vi "GEN_User Login Verify.vi"(8 "error in":errorcluster caption="错误输入（无错误）", 11 "User Archives":T1={"User Archives"=[{"User Name"="Admin", "Code"="123456", "Ability"=enum."Administrator", "Last Log Time"=timestamp(3476160307.20119 s since 1904-01-01)}, {"User Name"="Liusj", "Code"="123456", "Ability"=enum."Operator", "Last Log Time"=timestamp(3476160734.0536046 s since 1904-01-01)}], "Current User"=-1}) -> (0 "error out":errorcluster caption="错误输出", 1 "User Exist?":bool, 2 "User Archives out":T1={"User Archives"=[{"User Name"="Admin", "Code"="123456", "Ability"=enum."Administrator", "Last Log Time"=timestamp(3476160307.20119 s since 1904-01-01)}, {"User Name"="Liusj", "Code"="123456", "Ability"=enum."Operator", "Last Log Time"=timestamp(3476160734.0536046 s since 1904-01-01)}], "Current User"=-1}, 4 "Cancel?":bool)   [LabVIEW 2016]
uses:
  User Login_Archives Data Structure.ctl
panel:
  in  "Cancel Login":bool
  in  "User Login":bool
  in  "Code":string caption="密  码"
  in  "User Name":string="Admin" caption="用户名"
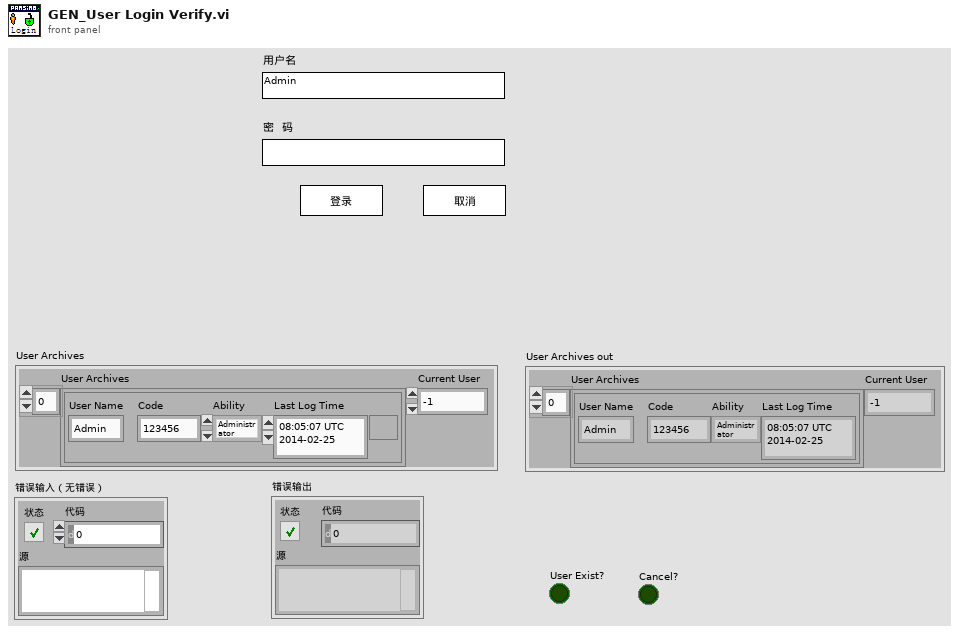
[diagram p1: front panel]
types:
  T1 = typedef "User Login_Archives Data Structure.ctl" = cluster{"User Archives":cluster{"User Name":string, "Code":string, "Ability":enum16{"Administrator", "Operator"}, "Last Log Time":timestamp}[], "Current User":i32}
  T2 = enum32{"Invalid", "Standard", "Closed", "Hidden", "Minimized", "Maximized"}
  T3 = cluster{"User Name":string, "Code":string, "Ability":enum16{"Administrator", "Operator"}, "Last Log Time":timestamp}[]
  T4 = cluster{"User Name":string, "Code":string, "Ability":enum16{"Administrator", "Operator"}, "Last Log Time":timestamp}
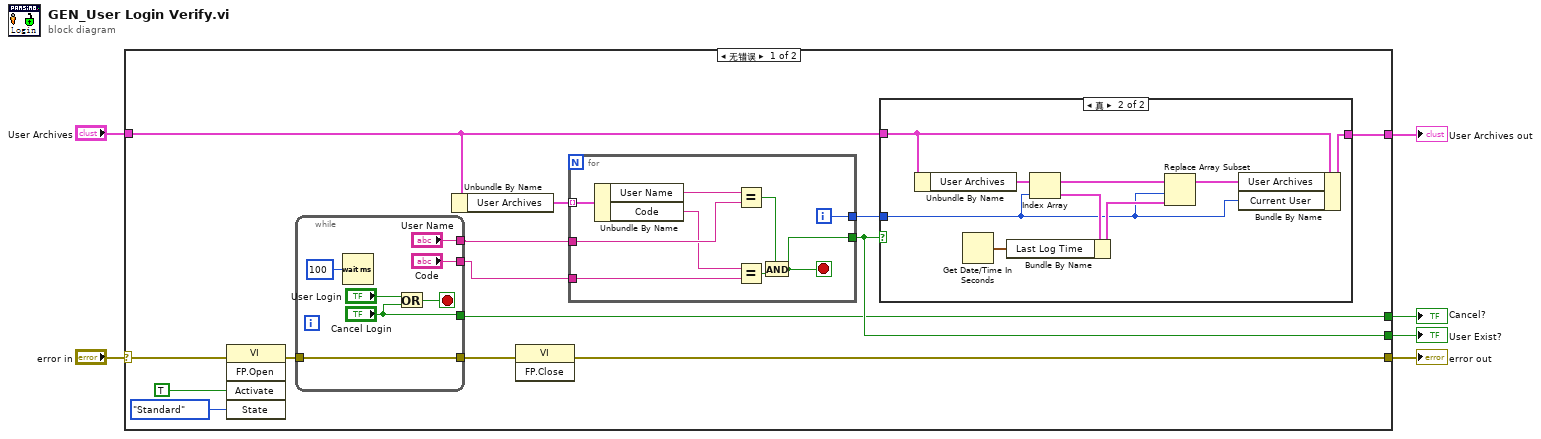
[diagram p0: block diagram]
diagram:
  n1 = case shown="无错误" "error in" {
    selector: "error in" -> [w13 w46]
    tunnel: [w19 _] -> w6
    tunnel: "User Archives" -> [w18 w47]
    tunnel: [w16 w47] -> w4
    tunnel: [w7 w46] -> w2
    tunnel: [w12 _] -> w1
    frame No Error {
      n2 = invoke class="VI" method="FP.Open"(error in=w13, "Activate"=TRUE ("激活？"), "State"=T2."Standard" ("状态")) -> (error out=w9:errorcluster)  [unwired: 2 in, 4 out]
      n3 = while {
        tunnel: ["User Name"] -> w15
        tunnel: ["Code"] -> w14
        tunnel: ["Cancel Login"] -> w12
        tunnel: w9 -> [w21]
        tunnel: [w21] -> w8
        stop <- w24 stop-if-true
        n4 = Wait (ms) ("等待(ms)")(milliseconds to wait=u32 100 ("等待时间（毫秒）")) -> ()  [unwired: 1 out]
        n5 = Or(x="User Login", y="Cancel Login") -> (x .or. y?=w24:bool)
      }
      n6 = Unbundle By Name(w18) -> ("User Archives"=w20:T3)
      n7 = invoke class="VI" method="FP.Close"(error in=w8) -> (error out=w7:errorcluster)  [unwired: 2 in, 2 out]
      n8 = for {
        tunnel: w15 -> [w43]
        tunnel: w14 -> [w41]
        tunnel: w20 -> [w45] mode=indexing
        tunnel: [w38] -> w19
        tunnel: [w37] -> w17
        i -> [w37]
        stop <- w38 stop-if-true
        n9 = Unbundle By Name(w45) -> ("User Name"=w44:string, "Code"=w42:string)
        n10 = Equal?(x=w44, y=w43) -> (x = y?=w40:bool)
        n11 = Equal?(x=w42, y=w41) -> (x = y?=w39:bool)
        n12 = And(x=w40, y=w39) -> (x .and. y?=w38:bool)
      }
      n13 = case shown="真" w19 {
        tunnel: w18 -> [w28 w35]
        tunnel: w17 -> [_ w29]
        tunnel: [w28 w36] -> w16
        frame False {
        }
        frame True {
          n14 = Unbundle By Name(w35) -> ("User Archives"=w32:T3)
          n15 = Get Date/Time In Seconds() -> (seconds since 1Jan1904=w33:timestamp)
          n16 = Index Array(array=w32, index=w29) -> (element=w34:T4)
          n17 = Bundle By Name(cluster=w34, "Last Log Time"=w33) -> (w31:T4)
          n18 = Replace Array Subset(array=w32, new element=w31, index=w29) -> (w30:T3)
          n19 = Bundle By Name(cluster=w35, "User Archives"=w30, "Current User"=w29) -> (w36:T1)
        }
      }
    }
    frame Error {
    }
  }
  "User Archives out" <- w4
  "User Exist?" <- w6
  "error out" <- w2
  "Cancel?" <- w1
